vi "WPI_CameraCountSameBufferNumber.vi"(8 "Duplicates":u32=10, 11 "Number":u32) -> (3 "Same":bool)   [LabVIEW 2017]
doc: "This VI counts the number of identical values in a sequence and returns a Boolean if greater than the limit. This is useful for identifying a stalled video session"
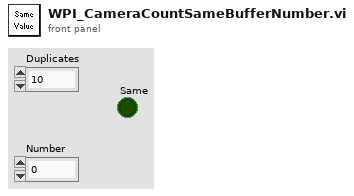
[diagram p1: front panel]
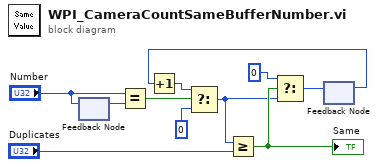
[diagram p0: block diagram]
diagram:
  n1 = feedback #1() -> (w10:u32)  [unwired: 1 in]
  n2 = feedback-in #1("Number") -> ()
  n3 = Equal?(x="Number", y=w10) -> (x = y?=w9:bool)
  n4 = feedback #2() -> (w8:i32)  [unwired: 1 in]
  n5 = Increment(x=w8) -> (x+1=w7:i32)
  n6 = Select(t=w7, s=w9, f=0) -> (s? t:f=w3:i32)
  n7 = Greater Or Equal?(x=w3, y="Duplicates") -> (x >= y?=w4:bool)
  "Same" <- w4
  n8 = Select(t=0, s=w4, f=w3) -> (s? t:f=w1:i32)
  n9 = feedback-in #2(w1) -> ()
